vi "Drive Away from Obstacle.vi"(4 "angle":dbl, 5 "max reverse velocity (m/s)":dbl, 6 "Find":bool, 7 "max angular velocity (rad/s)":dbl=1.0, 8 "error in (no error)":errorcluster, 9 "Tank1":dbl[](array[numeric]), 10 "Tank2":dbl[](array[numeric]), 11 "gap":T1) -> (0 "error out":errorcluster, 2 "steering frame velocity":dbl[](array[numeric]))   [LabVIEW 2012]
doc: "Sets the steering frame velocity so that the robot moves in reverse and rotates towards the gap."
uses:
  <vilib>/robotics/Obstacle Avoidance/Simple Vector Field Histogram/Gap Description.ctl
  <vilib>/imath/engines/lvmath2/RunTimeEngine/ErrorHandling/NIMS_Finalize Error.vi
  <vilib>/robotics/Obstacle Avoidance/Simple Vector Field Histogram/NI_Robotics_Simple Vector Field Histogram.lvlib
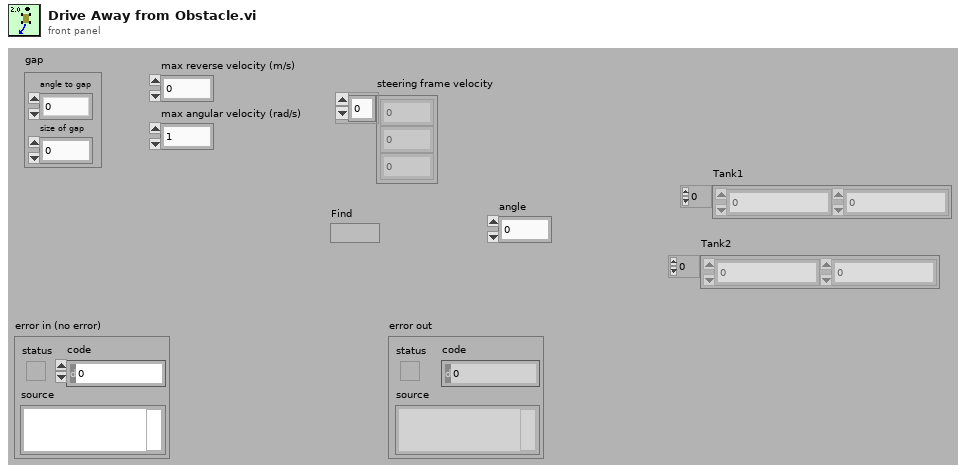
[diagram p1: front panel]
types:
  T1 = typedef "NI_Robotics_Simple Vector Field Histogram.lvlib/Gap Description.ctl" = cluster{"angle to gap":dbl, "size of gap":dbl}
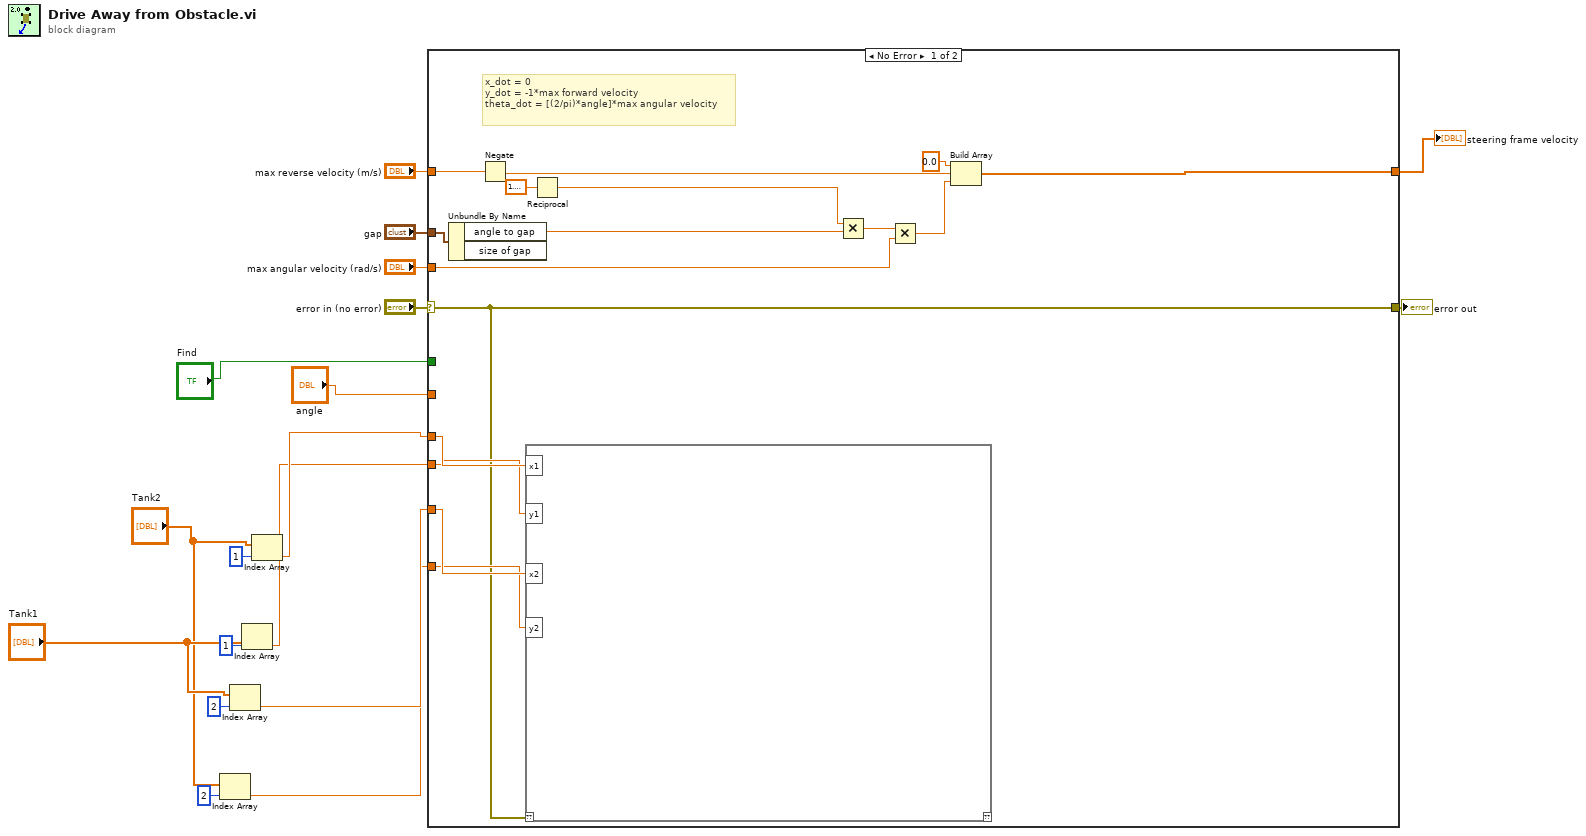
[diagram p0: block diagram]
diagram:
  n1 = Index Array(array="Tank2", index=2) -> (element=w5:dbl)
  n2 = Index Array(array="Tank1", index=2) -> (element=w6:dbl)
  n3 = Index Array(array="Tank1", index=1) -> (element=w7:dbl)
  n4 = Index Array(array="Tank2", index=1) -> (element=w8:dbl)
  n5 = case shown="No Error" "error in (no error)" {
    selector: "error in (no error)" -> [w20 w45]
    tunnel: "gap" -> [w34 _]
    tunnel: [w20 w45] -> w16
    tunnel: "max reverse velocity (m/s)" -> [w31 _]
    tunnel: "max angular velocity (rad/s)" -> [w26 _]
    tunnel: [w32 _] -> w13
    tunnel: w8 -> [w24 _]
    tunnel: w7 -> [w23 _]
    tunnel: w6 -> [w22 _]
    tunnel: w5 -> [w21 _]
    tunnel: "Find" -> [_ _]
    tunnel: "angle" -> [_ _]
    frame No Error {
      # "x_dot = 0\ny_dot = -1*max forward velocity\ntheta_dot = [(2/pi)*angle]*max angular velocity"
      n6 = Unbundle By Name(w34) -> ("angle to gap"=w19:dbl)  [unwired: 1 out]
      n7 = Negate(x=w31) -> (-x=w30:dbl)
      n8 = mathscript code="1"("??"=w20, "x1"=w24, "y1"=w23, "x2"=w22, "y2"=w21) -> ()  [unwired: 1 out]
      n9 = Reciprocal(x=1.5707963267948966) -> (1/x=w28:dbl)
      n10 = Multiply(x=w28, y=w19) -> (x*y=w27:dbl)
      n11 = Multiply(x=w27, y=w26) -> (x*y=w25:dbl)
      n12 = Build Array(0.0 ("element"), w30, w25) -> (w32:dbl[])
    }
    frame Error {
    }
  }
  "error out" <- w16
  "steering frame velocity" <- w13
